vi "XLP80_CAN_GetWriteIndex.vi"(6 "Init":bool, 10 "CAN Write Items":T1) -> (2 "Index":i32)   [LabVIEW 2021]
uses:
  XLP80_FGlob/1886_FGlob_TDefEnumCANWriteItems.ctl
  XLP80_Globals/XLP80_Globals_Status.vi
  XLP80_Globals/Globals_Settings_XLP80.vi
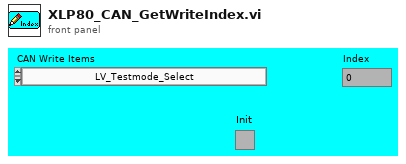
[diagram p1: front panel]
types:
  T1 = typedef "1886_FGlob_TDefEnumCANWriteItems.ctl" = enum16{"LV_Testmode_Select", "LV_A_71_Current_Out_Set", "LV_A_71_Voltage_In_Set", "LV_A_71_Voltage_Out_Set", "LV_H_51_STK_CellVoltages_Enable", "S80_BP_s_Taster_Start_Status"}
  T2 = typedef "XLP80_Action_TDefEnumControl.ctl" = enum16{"Testmode_A", "Testmode_B"}
  T3 = cluster{"Signal Name":string[], "Description":string[], "Unit":string[], "Default":dbl[], "Min":dbl[], "Max":dbl[], "TestmodeA":bool[], "LogEnable":bool[]}
  T4 = cluster{"Signal Name":string[], "Description":string[], "Unit":string[], "Default":dbl[], "Min":dbl[], "Max":dbl[], "Preconditions":bool[], "HV & Software":bool[], "Basis Funktion":bool[], "Power Management":bool[], "OperationMode":bool[], "Shutdown":bool[], "Alarm":bool[], "LogEnable":bool[]}
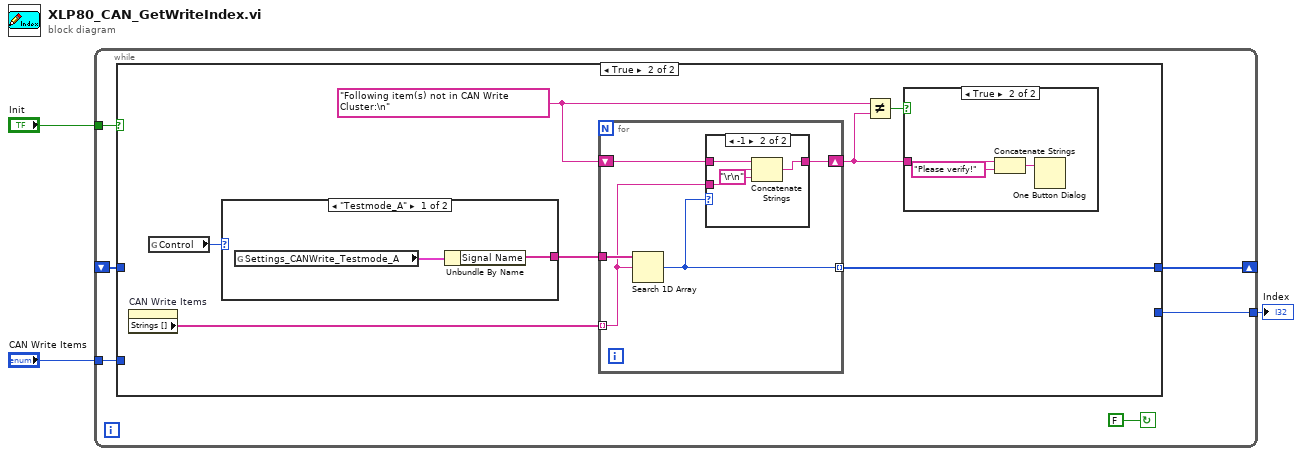
[diagram p0: block diagram]
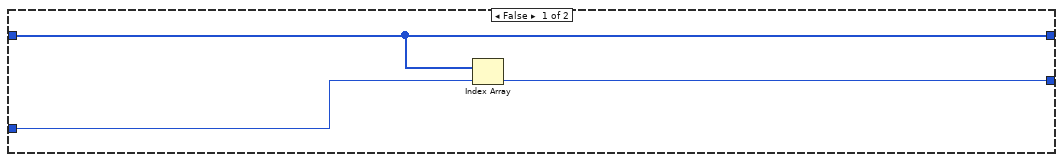
[diagram p2: hidden frame]
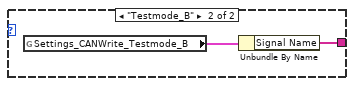
[diagram p5: hidden frame]
diagram:
  n1 = while {
    tunnel: "Init" -> [w8]
    tunnel: "CAN Write Items" -> [w7]
    shift-right: [w6] -> _
    shift-left: _ -> [w5]
    tunnel: [w4] -> w1
    stop <- FALSE continue-if-true
    n2 = case shown="True" w8 {
      tunnel: w7 -> [w11 _]
      tunnel: [w12 w17] -> w6
      tunnel: w5 -> [w12 _]
      tunnel: [w10 _] -> w4
      frame False {
        n3 = Index Array(array=w12, index=w11) -> (element=w10:i32)
      }
      frame True {
        w14 = "Following item(s) not in CAN Write Cluster:\n"
        n4 = property on="CAN Write Items" class="Enum (strict)"() -> ("Strings []"=w16:string[])  [unwired: 2 in, 2 out]
        n5 = global read "XLP80_Globals_Status.vi" "Control"() -> (w19:T2)
        n6 = case shown="\"Testmode_A\"" w19 {
          tunnel: [w33 w35] -> w18
          frame "Testmode_A" {
            n7 = global read "Globals_Settings_XLP80.vi" "Settings_CANWrite_Testmode_A"() -> (w34:T3)
            n8 = Unbundle By Name(w34) -> ("Signal Name"=w33:string[])
          }
          frame "Testmode_B" {
            n9 = global read "Globals_Settings_XLP80.vi" "Settings_CANWrite_Testmode_B"() -> (w36:T4)
            n10 = Unbundle By Name(w36) -> ("Signal Name"=w35:string[])
          }
        }
        n11 = for {
          tunnel: w18 -> [w27]
          tunnel: [w26] -> w17 mode=indexing
          tunnel: w16 -> [w25] mode=indexing
          shift-right: [w23] -> w13
          shift-left: w14 -> [w24]
          n12 = Search 1D Array(1D array=w27, element=w25) -> (index of element=w26:i32)  [unwired: 1 in]
          n13 = case shown="-1" w26 {
            tunnel: w25 -> [_ w31]
            tunnel: w24 -> [w28 w32]
            tunnel: [w28 w29] -> w23
            frame Default {
            }
            frame -1 {
              n14 = Concatenate Strings(w32, w31, "\r\n") -> (w29:string)
            }
          }
        }
        n15 = Not Equal?(x=w14, y=w13) -> (x != y?=w15:bool)
        n16 = case shown="True" w15 {
          tunnel: w13 -> [_ w22]
          frame False {
          }
          frame True {
            n17 = Concatenate Strings(w22, "Please verify!" ("string")) -> (w21:string)
            n18 = One Button Dialog(message=w21) -> ()  [unwired: 1 in, 1 out]
          }
        }
      }
    }
  }
  "Index" <- w1
